vi "StartActor.vi"(6 "Reference":refnum<vi>, 8 "ErrorIn":errorcluster, 11 "YActorIn":refnum<class "YActor.lvclass">) -> (0 "ErrorOut":errorcluster)   [LabVIEW 2021, in "YActor.lvclass"]
uses:
  YActor.lvclass
  YActor.lvclass/YActor.ctl
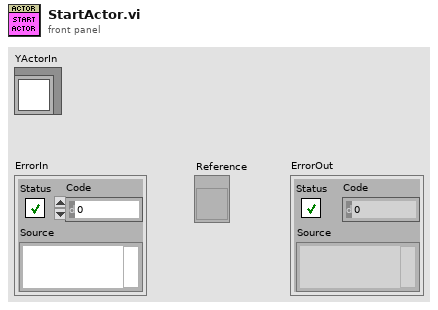
[diagram p1: front panel]
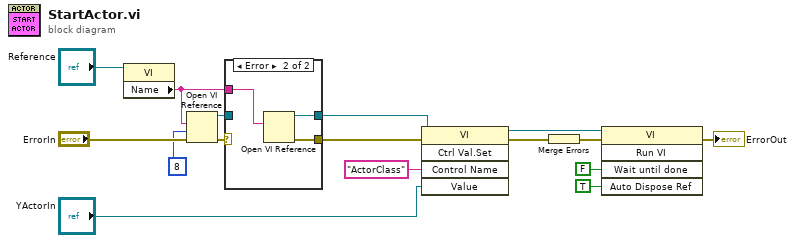
[diagram p0: block diagram]
diagram:
  n1 = property class="VI"(reference="Reference") -> ("Name"=w4:string)  [unwired: 1 in, 2 out]
  n2 = Open VI Reference(vi path=w4, options=8, error in (no error)="ErrorIn") -> (vi reference=w3:refnum<vi>, error out=w13:errorcluster)  [unwired: 3 in]
  n3 = case shown="Error" w13 {
    selector: w13 -> [w18 _]
    tunnel: w4 -> [_ w20]
    tunnel: [w18 w21] -> w12
    tunnel: [w17 w19] -> w1
    tunnel: w3 -> [w17 _]
    frame No Error {
    }
    frame Error {
      n4 = Open VI Reference(vi path=w20) -> (vi reference=w19:refnum<vi>, error out=w21:errorcluster)  [unwired: 5 in]
    }
  }
  n5 = invoke class="VI" method="Ctrl Val.Set"(reference=w1, error in=w12, "Control Name"="ActorClass", "Value"="YActorIn") -> (reference out=w9:refnum<vi>, error out=w16:errorcluster)  [unwired: 1 in, 3 out]
  n6 = Merge Errors(w16) -> (w11:errorcluster)
  n7 = invoke class="VI" method="Run VI"(reference=w9, error in=w11, "Wait until done"=FALSE ("Wait Until Done"), "Auto Dispose Ref"=TRUE ("Auto Dispose Reference")) -> (error out=→"ErrorOut":errorcluster)  [unwired: 1 in, 4 out]
